vi "Write Float Register.vi"(7 "PDU Address 32-bit Float":T1 items=["FSetpoint"=41240, "Capacity 0%"=41392, "Counter limit (Float)"=59416, "PID-Kp"=62120, "PID-Ti"=62128, "PID-Td"=62136, "Dynamic display factor"=62728, "Static display factor"=62736, "Exponential smoothing"=62752], 8 "error in":errorcluster, 10 "Value":sgl, 11 "MB_TCP session in":refnum<class "MB_Master_TCP.lvclass">) -> (0 "error out":errorcluster, 3 "MB session out":refnum<class "MB_Master_TCP.lvclass">)   [LabVIEW 2024, in "Bronkhorst Flexi-Flow ModbusTCP API.lvlib"]
uses:
  Bronkhorst Flexi-Flow ModbusTCP API.lvlib
  <vilib>/Plasmionique/MB Master/MB_Master_TCP/MB_Master_TCP.lvclass
  C:/Program Files/National Instruments/LabVIEW 2025/vi.lib/Plasmionique/MB Master/MB_Master/MB_Master.lvclass
  PDU Address Float 32-bit Params--ring.ctl
  <vilib>/Plasmionique/MB Master/MB Master.lvlib
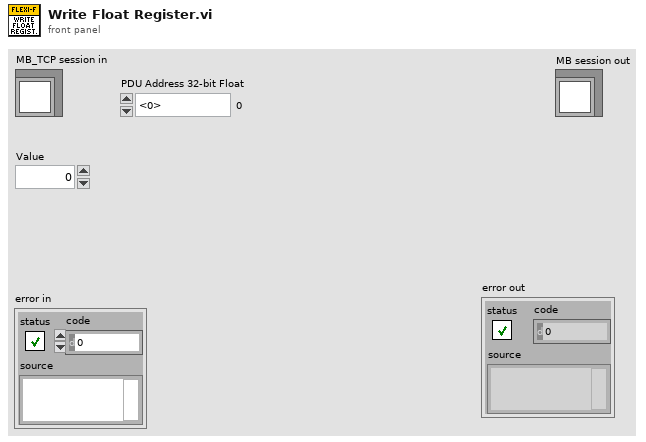
[diagram p1: front panel]
types:
  T1 = typedef "Bronkhorst Flexi-Flow ModbusTCP API.lvlib/PDU Address Float 32-bit Params--ring.ctl" = u16
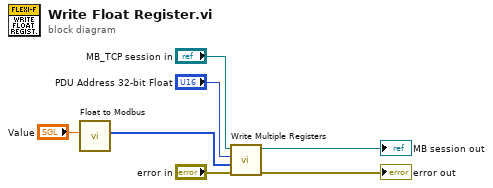
[diagram p0: block diagram]
diagram:
  n1 = call "Float to Modbus.vi"("32-Bit Float"="Value") -> ("Registers"=w1:u16[])  [unwired: 10 in]
  n2 = call <vilib>:"Write Multiple Registers.vi"("error in (no error)"="error in", "values"=w1, "starting address"="PDU Address 32-bit Float", "MB session in"="MB_TCP session in") -> ("error out"=→"error out":errorcluster, "MB session out"=→"MB session out":refnum<class "MB_Master_TCP.lvclass">)  [unwired: 6 in]
